vi "Frame.Get.Size.vi"(11 "Parameters":T1[](array[typedef]) {"Byte Order" items=["Little Endian", "Big Endian"]; "Data Type" items=["Signed", "Unsigned", "IEEE Float"]}) -> (3 "Bytes":u32)   [LabVIEW 2019, in "Diagnostics Addon Shared.lvlib"]
uses:
  Diagnostics Addon Shared.lvlib
  Types/Signal.ctl
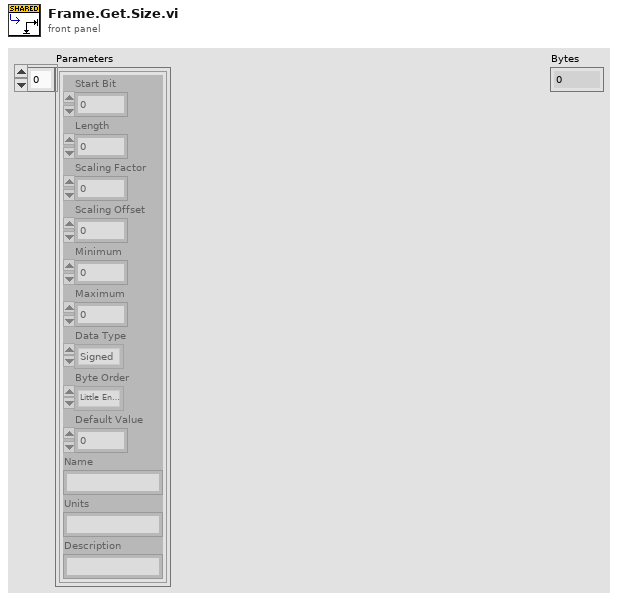
[diagram p1: front panel]
types:
  T1 = typedef "Diagnostics Addon Shared.lvlib/Signal.ctl" = cluster{"Start Bit":u32, "Length":u32, "Scaling Factor":dbl, "Scaling Offset":dbl, "Minimum":dbl, "Maximum":dbl, "Data Type":u32, "Byte Order":u32, "Default Value":dbl, "Name":string, "Units":string, "Description":string}
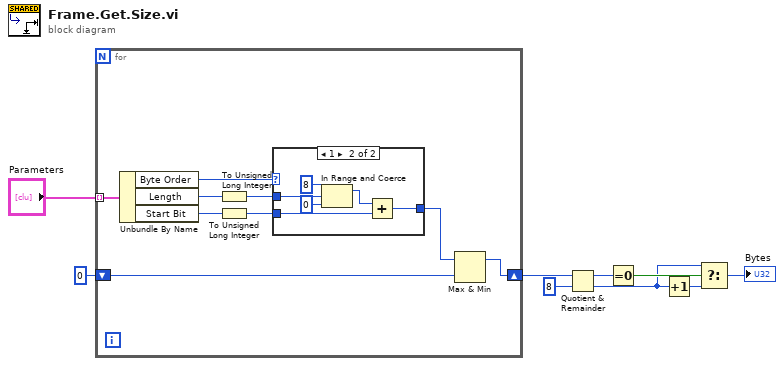
[diagram p0: block diagram]
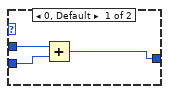
[diagram p2: hidden frame]
diagram:
  n1 = for {
    tunnel: "Parameters" -> [w18] mode=indexing
    shift-right: [w16] -> w7
    shift-left: u16 0 -> [w17]
    n2 = Unbundle By Name(w18) -> ("Byte Order"=w15:u32, "Length"=w14:u32, "Start Bit"=w13:u32)
    n3 = To Unsigned Long Integer(number=w14) -> (unsigned 32bit integer=w10:u32)
    n4 = To Unsigned Long Integer(number=w13) -> (unsigned 32bit integer=w11:u32)
    n5 = case shown="1" w15 {
      tunnel: w10 -> [w21 w26]
      tunnel: w11 -> [w20 w27]
      tunnel: [w19 w22] -> w12
      frame 0, Default {
        n6 = Add(x=w21, y=w20) -> (x+y=w19:u32)
      }
      frame 1 {
        n7 = In Range and Coerce(upper limit=u32 8, x=w26, lower limit=u32 0) -> (coerced(x)=w23:u32)  [unwired: 1 out]
        n8 = Add(x=w23, y=w27) -> (x+y=w22:u32)
      }
    }
    n9 = Max & Min(x=w12, y=w17) -> (max(x,y)=w16:u32)  [unwired: 1 out]
  }
  n10 = Quotient & Remainder(x=w7, y=u32 8) -> (x-y*floor(x/y)=w5:u32, floor(x/y)=w3:u32)
  n11 = Equal To 0?(x=w5) -> (x = 0?=w4:bool)
  n12 = Increment(x=w3) -> (x+1=w2:u32)
  n13 = Select(t=w3, s=w4, f=w2) -> (s? t:f=→"Bytes":u32)
